vi "ArrayAsStringArray.vi"(8 "error in (no error)":errorcluster, 11 "Array Parameter":string="\n      <array>\n  <data>\r<value><double>0.000000</double></value>\r<value><double>1.175571</double></value>\r<value><double>1.902113</double></value>\r<value><double>1.902113</double></value>\r<value><double>1.175571</double></value>\r<value><double>0.000000</double></value>\r<value><double>-1.175571</double></value>\r<value><double>-1.902113</double></value>\r<value><double>-1.902113</double></value>\r<value><double>-1.175571</double></value>\r<value><double>0.000000</double></value>\r<value><double>1.175571</double></value>\r<value><double>1.902113</double></value>\r<value><double>1.902113</double></value>\r<value><double>1.175571</double></value>\r<value><double>0.000000</double></value>\r<value><double>-1.175571</double></value>\r<value><double>-1.902113</double></value>\r<value><double>-1.902113</double></value>\r<value><double>-1.175571</double></value>\r<value><double>0.000000</double></value>\r<value><double>1.175571</double></value>\r<value><double>1.902113</double></value>\r<value><double>1.902113</double></value>\r<value><double>1.175571</double></value>\r<value><double>0.000000</double></value>\r<value><double>-1.175571</double></value>\r<value><double>-1.902113</double></value>\r<value><double>-1.902113</double></value>\r<value><double>-1.175571</double></value>\r<value><double>0.000000</double></value>\r<value><double>1.175571</double></value>\r<value><double>1.902113</double></value>\r<value><double>1.902113</double></value>\r<value><double>1.175571</double></value>\r<value><double>0.000000</double></value>\r<value><double>-1.175571</double></value>\r<value><double>-1.902113</double></value>\r<value><double>-1.902113</double></value>\r<value><double>-1.175571</double></value>\r<value><double>0.000000</double></value>\r<value><double>1.175571</double></value>\r<value><double>1.902113</double></value>\r<value><double>1.902113</double></value>\r<value><double>1.175571</double></value>\r<value><double>0.000000</double></value>\r<value><double>-1.175571</double></value>\r<value><double>-1.902113</double></value>\r<value><double>-1.902113</double></value>\r<value><double>-1.175571</double></value>\r<value><double>0.000000</double></value>\r<value><double>1.175571</double></value>\r<value><double>1.902113</double></value>\r<value><double>1.902113</double></value>\r<value><double>1.175571</double></value>\r<value><double>0.000000</double></value>\r<value><double>-1.175571</double></value>\r<value><double>-1.902113</double></value>\r<value><double>-1.902113</double></value>\r<value><double>-1.175571</double></value>\r<value><double>0.000000</double></value>\r<value><double>1.175571</double></value>\r<value><double>1.902113</double></value>\r<value><double>1.902113</double></value>\r<value><double>1.175571</double></value>\r<value><double>0.000000</double></value>\r<value><double>-1.175571</double></value>\r<value><double>-1.902113</double></value>\r<value><double>-1.902113</double></value>\r<value><double>-1.175571</double></value>\r<value><double>0.000000</double></value>\r<value><double>1.175571</double></value>\r<value><double>1.902113</double></value>\r<value><double>1.902113</double></value>\r<value><double>1.175571</double></value>\r<value><double>0.000000</double></value>\r<value><double>-1.175571</double></value>\r<value><double>-1.902113</double></value>\r<value><double>-1.902113</double></value>\r<value><double>-1.175571</double></value>\r<value><double>0.000000</double></value>\r<value><double>1.175571</double></value>\r<value><double>1.902113</double></value>\r<value><double>1.902113</double></value>\r<value><double>1.175571</double></value>\r<value><double>0.000000</double></value>\r<value><double>-1.175571</double></value>\r<value><double>-1.902113</double></value>\r<value><double>-1.902113</double></value>\r<value><double>-1.175571</double></value>\r<value><double>0.000000</double></value>\r<value><double>1.175571</double></value>\r<value><double>1.902113</double></value>\r<value><double>1.902113</double></value>\r<value><double>1.175571</double></value>\r<value><double>0.000000</double></value>\r<value><double>-1.175571</double></value>\r<value><double>-1.902113</double></value>\r<value><double>-1.902113</double></value>\r<value><double>-1.175571</double></value>\r<value><double>0.000000</double></value>\r<value><double>1.175571</double></value>\r<value><double>1.902113</double></value>\r<value><double>1.902113</double></value>\r<value><double>1.175571</double></value>\r<value><double>0.000000</double></value>\r<value><double>-1.175571</double></value>\r<value><double>-1.902113</double></value>\r<value><double>-1.902113</double></value>\r<value><double>-1.175571</double></value>\r<value><double>0.000000</double></value>\r<value><double>1.175571</double></value>\r<value><double>1.902113</double></value>\r<value><double>1.902113</double></value>\r<value><double>1.175571</double></value>\r<value><double>0.000000</double></value>\r<value><double>-1.175571</double></value>\r<value><double>-1.902113</double></value>\r<value><double>-1.902113</double></value>\r<value><double>-1.175571</double></value>\r<value><double>0.000000</double></value>\r<value><double>1.175571</double></value>\r<value><double>1.902113</double></value>\r<value><double>1.902113</double></value>\r<value><double>1.175571</double></value>\r<value><double>0.000000</double></value>\r<value><double>-1.175571</double></value>\r<value><double>-1.902113</double></value>\n  </data>\n</array>\n    ") -> (0 "error out":errorcluster, 3 "ArrayAsValues":string[](array[string]))   [LabVIEW 2009]
doc: "Convert an XML-RPC formatted array to a LV array of XML_RPC formatted values"
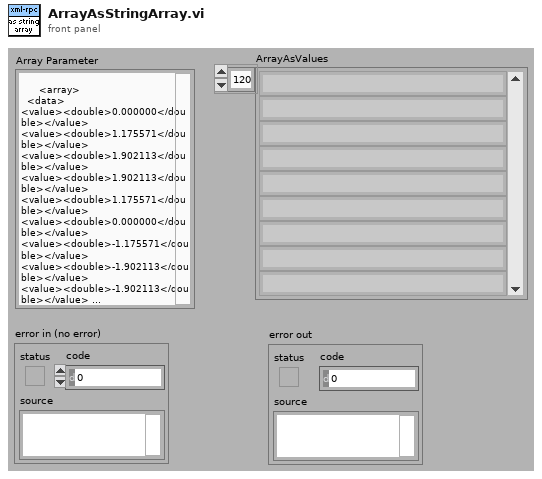
[diagram p1: front panel]
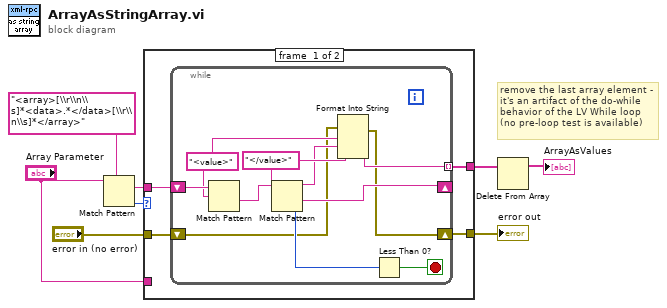
[diagram p0: block diagram]
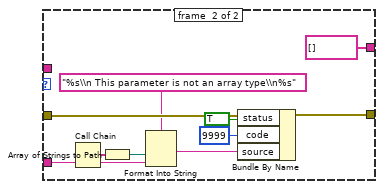
[diagram p2: hidden frame]
diagram:
  # "remove the last array element - it's an artifact of the do-while behavior of the LV While loop (no pre-loop test is available)"
  n1 = Match Pattern(string="Array Parameter", regular expression="<array>[\\r\\n\\s]*<data>.*</data>[\\r\\n\\s]*</array>") -> (match substring=w3:string, offset past match=w7:i32)  [unwired: 1 in, 2 out]
  n2 = case shown="0, Default" w7 {
    tunnel: "error in (no error)" -> [w10 w32]
    tunnel: [w9 w31] -> w5
    tunnel: "Array Parameter" -> [_ w26]
    tunnel: w3 -> [w12 _]
    tunnel: [w11 string[] []] -> w2
    frame #0 {
      n3 = while {
        shift-right: [w20] -> _
        shift-left: w12 -> [w23]
        tunnel: [w17] -> w11 mode=indexing
        shift-right: [w13] -> w9
        shift-left: w10 -> [w14]
        stop <- w22 stop-if-true
        w16 = "</value>" ("regular expression")
        w18 = "<value>" ("regular expression")
        n4 = Match Pattern(string=w23, regular expression=w18) -> (after substring=w21:string)  [unwired: 1 in, 3 out]
        n5 = Match Pattern(string=w21, regular expression=w16) -> (before substring=w15:string, after substring=w20:string, offset past match=w19:i32)  [unwired: 1 in, 1 out]
        n6 = Format Into String(error in=w14, w18, w15, w16) -> (resulting string=w17:string, error out=w13:errorcluster)  [unwired: 2 in]
        n7 = Less Than 0?(x=w19) -> (x < 0?=w22:bool)
      }
    }
    frame #1 {
      n8 = Call Chain() -> (call chain=w33:string[])
      n9 = Array of Strings to Path(0:w33) -> (2:w28:path)  [unwired: 1 in]
      n10 = Format Into String(format string="%s\\n This parameter is not an array type\\n%s", w28, w26) -> (resulting string=w27:string)  [unwired: 2 in, 1 out]
      n11 = Bundle By Name(cluster=w32, "status"=TRUE, "code"=9999, "source"=w27) -> (w31:errorcluster)
    }
  }
  "error out" <- w5
  n12 = Delete From Array(array=w2) -> (array with subset deleted=→"ArrayAsValues":string[])  [unwired: 2 in, 1 out]
